vi "SubTest.vi"(8 "error in (no error)":errorcluster) -> (0 "error out":errorcluster)   [LabVIEW 2017]
uses:
  <vilib>/addons/_JKI Toolkits/Caraya/classes/Test/Test.lvclass
  <vilib>/addons/_JKI Toolkits/Caraya/classes/Assert/Assert.lvclass
  <vilib>/addons/_JKI Toolkits/Caraya/classes/Assert/Assert True.vi
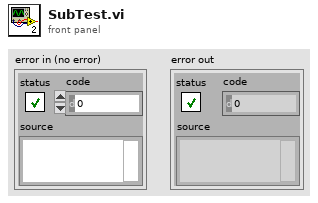
[diagram p1: front panel]
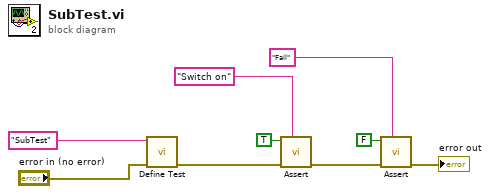
[diagram p0: block diagram]
diagram:
  n1 = call <vilib>:"Define Test.vi"("error in (no error)"="error in (no error)", "Label (VI Title)"="SubTest") -> ("error out"=w7:errorcluster)  [unwired: 8 in, 1 out]
  n2 = call-poly <vilib>:"Assert.vi"("Label"="Switch on", "error in (no error)"=w7, "True?"=TRUE) -> ("error out"=w2:errorcluster)  [unwired: 7 in, 1 out]
  n3 = call-poly <vilib>:"Assert.vi"("Label"="Fail", "error in (no error)"=w2, "True?"=FALSE) -> ("error out"=→"error out":errorcluster)  [unwired: 7 in, 1 out]
